vi "target_b2g2.vi"   [LabVIEW 2011]
uses:
  Output - Cluster b2g1.ctl
  Output - Cluster b2g2.ctl
  Input - Cluster b2g2.ctl
  <vilib>/Platform/TimedLoop/XDataNode/timing_clust.ctl
  <vilib>/Platform/TimedLoop/XDataNode/nitl_modes.ctl
  <vilib>/Platform/TimedLoop/XDataNode/wakeup.ctl
  <vilib>/Utility/error.llb/DialogType.ctl
  <vilib>/Platform/TimedLoop/XDataNode/XDataNode.xnode
  <vilib>/Platform/TimedLoop/XDataNode/XDNodeRunTimeDep.lvlib
panel:
  # "The Network Variable Engine and Variable Client Support must be installed on the RT target\nfor this application to function properly. If the Network Variable Engine is not supported on\nthe target (e.g.  FP-2000 with <32MB of RAM), open the project and move the variable library\nto My Computer in the project. Doing this will deploy the variables to localhost but\nwill still require that Variable Client Support be installed on the RT target."
types:
  T1 = typedef "XDNodeRunTimeDep.lvlib/timing_clust.ctl" = cluster{"Expected End [f-1]":u64, "Actual End [f-1]":u64, "Finished Late? [f-1]":bool, "Expected End [i-1]":u64, "Actual End [i-1]":u64, "Finished Late? [i-1]":bool, "Expected Start [i]":u64, "Actual Start [i]":u64, "Expected Start [f]":u64, "Actual Start [f]":u64, "Source Name":string, "Structure Name":string, "Period":i64, "Deadline":i64, "Offset":i64, "Start":i64, "Priority":i32, "Timeout":i32, "Mode":T2, "Wakeup Reason":T3, "Error":errorcluster, "Source Type":string, "Secondary Source Type":string, "Global End Time":u64, "Global Start Time":u64, "Frame Duration":u64, "Iteration Duration":u64, "Assigned CPU":i32, "I/O Scan Engine Mode":u32}
  T2 = typedef "XDNodeRunTimeDep.lvlib/nitl_modes.ctl" = enum32{"No Change", "Process missed periods, maintain original phase", "Discard missed periods, maintain original phase", "Process missed periods, ignore original phase", "Discard missed periods, ignore original phase"}
  T3 = typedef "XDNodeRunTimeDep.lvlib/wakeup.ctl" = enum32{"Normal", "Aborted", "Asynchronous wakeup", "Timing source error", "Timed loop error", "Timeout"}
  T4 = typedef "Output - Cluster b2g1.ctl" = cluster{"DFS-1 [dl]":u64, "FS-3 [l]":dbl, "DFS-1 [l/min]":dbl, "DS-1 [bar]":dbl, "V-10 ZU":bool, "V-14 ZU":bool, "FS-1 [l]":dbl, "FS-2 [l]":dbl, "TS-4 [°C]":dbl, "HS-1":bool, "V-13 [%]":u8, "V-15 [%]":u8, "P-4 [%]":u8, "P-5 [%]":u8, "Dosierung":bool, "MR Max Füllstand":bool, "MR Min Füllstand":bool, "Dosiermenge [l]":sgl, "V-14 AUF":bool, "V-10 AUF":bool, "T-1 Max Füllstand":bool, "T-1 Min Füllstand":bool, "T-2 Max Füllstand":bool, "T-2 Min Füllstand":bool, "pHS-1 [pH]":dbl, "P-4 RUN":bool, "P-5 RUN ":bool, "V-33 AUF":bool, "V-33 ZU":bool, "V-34 AUF":bool, "V-34 ZU":bool, "P-4 ERR":bool, "P-5 ERR":bool, "TS-5 [°C]":dbl, "TS-6 [°C]":dbl, "P-9 RUN":bool}
  T5 = cluster{"clusterb2g1":bool, "STOP":bool, "data - network -  b2g1":refnum<k21>, "shared variable refnum out":refnum<k21>}
  T6 = typedef "Output - Cluster b2g2.ctl" = cluster{"DFS-1 [dl]":u64, "FS-3 [l]":dbl, "DFS-1 [l/min]":dbl, "DS-1 [bar]":dbl, "V-10 ZU":bool, "V-14 ZU":bool, "FS-1 [l]":dbl, "FS-2 [l]":dbl, "TS-4 [°C]":dbl, "HS-1":bool, "V-13 [%]":u8, "V-15 [%]":u8, "P-4 [%]":u8, "Dosierung":bool, "MR Max Füllstand":bool, "MR Min Füllstand":bool, "Dosiermenge [l]":sgl, "V-14 AUF":bool, "V-10 AUF":bool, "T-1 Max Füllstand":bool, "T-1 Min Füllstand":bool, "T-2 Max Füllstand":bool, "T-2 Min Füllstand":bool, "pHS-1 [pH]":dbl, "P-4 RUN":bool, "V-33 AUF":bool, "V-33 ZU":bool, "V-34 AUF":bool, "V-34 ZU":bool, "P-4 ERR":bool, "TS-5 [°C]":dbl, "V-35 AUF":bool, "V-35 ZU":bool, "P-9 RUN":bool}
  T7 = cluster{"Durchflussregelung":dbl, "Temperaturregelung":bool, "STOP":bool, "Zirkulation":u64, "Dosierung Zeit":u64}
  T8 = typedef "Input - Cluster b2g2.ctl" = cluster{"V-13 [%]":u8, "V-15 [%]":u8, "Log-Target":bool, "P-4":bool, "P-4 Drehzahl [%]":u8, "Temperaturregelung":bool, "Überdruckregelung":bool, "Füllstandsregulierung":bool, "V-10":bool, "Log-Host":bool, "V-14":bool, "HS-1":bool, "Füllstand  P":sgl, "Füllstand I":sgl, "Füllstand D":sgl, "Füllstand Soll [l]":sgl, "Druck  P":sgl, "Druck I":sgl, "Druck D":sgl, "Druck Soll [bar]":sgl, "Temp Soll [°C]":sgl, "Dosierung":bool, "Dosiermenge [l]":sgl, "Dosiergeschw. [l/min]":sgl, "Tank":bool, "Hysterese [°C]":sgl, "MR Füllstandsüberwachung":bool, "Tank Füllstandsüberwachung":bool, "Log Target [ms]":u32, "Log Host [s]":u32, "Zirkulation EIN [min]":u8, "Zirkulation AUS [min]":u8, "Zirkulation":bool, "V-33":bool, "V-34":bool, "V-35":bool, "T1 Max Füllstand":bool, "T1 Min Füllstand":bool, "FS-1 [l]":sgl, "P-9":bool}
  T9 = typedef "DialogType.ctl" = u16
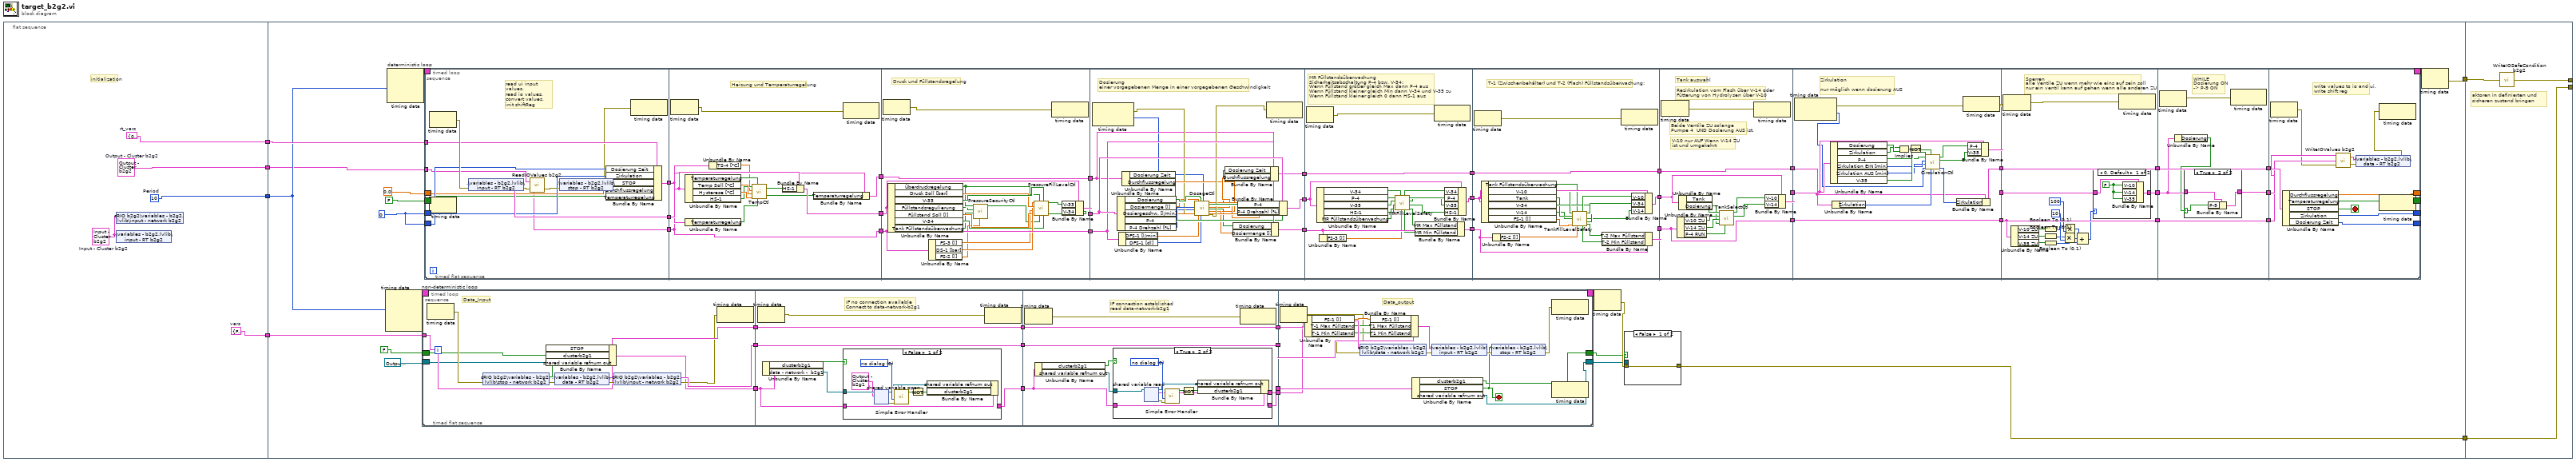
[diagram p0: block diagram]
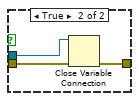
[diagram p2: hidden frame]
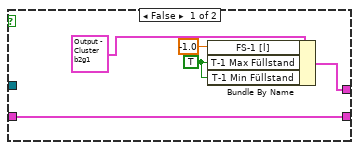
[diagram p4: hidden frame]
diagram:
  n1 = flat-sequence {
    tunnel: [w10] -> w6
    tunnel: [w9] -> w5
    tunnel: [w8] -> w4
    tunnel: [w7] -> w1
    tunnel: w6 -> [w23]
    tunnel: w5 -> [w22]
    tunnel: w4 -> [w21]
    tunnel: [w17] -> w3
    tunnel: [w20] -> w2
    tunnel: w1 -> [w16]
    tunnel: w3 -> [w441]
    tunnel: w2 -> [w440]
    tunnel: [w439] -> _
    tunnel: [w441] -> _
    frame #0 {
      w7 = T5 {"clusterb2g1"=FALSE, "STOP"=FALSE, "data - network -  b2g1"="ni.var.psp://10.27.40.24/variables - b2g1/data - network - b2g1", "shared variable refnum out"=""}  # vars
      w8 = T6 {"DFS-1 [dl]"=0, "FS-3 [l]"=0.0, "DFS-1 [l/min]"=0.0, "DS-1 [bar]"=0.0, "V-10 ZU"=FALSE, "V-14 ZU"=FALSE, "FS-1 [l]"=0.0, "FS-2 [l]"=0.0, "TS-4 [°C]"=0.0, "HS-1"=FALSE, "V-13 [%]"=0, "V-15 [%]"=0, "P-4 [%]"=0, "Dosierung"=FALSE, "MR Max Füllstand"=FALSE, "MR Min Füllstand"=FALSE, "Dosiermenge [l]"=0.0, "V-14 AUF"=FALSE, "V-10 AUF"=FALSE, "T-1 Max Füllstand"=FALSE, "T-1 Min Füllstand"=FALSE, "T-2 Max Füllstand"=FALSE, "T-2 Min Füllstand"=FALSE, "pHS-1 [pH]"=0.0, "P-4 RUN"=FALSE, "V-33 AUF"=FALSE, "V-33 ZU"=FALSE, "V-34 AUF"=FALSE, "V-34 ZU"=FALSE, "P-4 ERR"=FALSE, "TS-5 [°C]"=0.0, "V-35 AUF"=FALSE, "V-35 ZU"=FALSE, "P-9 RUN"=FALSE}  # Output - Cluster b2g2
      w10 = T7 {"Durchflussregelung"=0.0, "Temperaturregelung"=FALSE, "STOP"=FALSE, "Zirkulation"=0, "Dosierung Zeit"=0}  # rt_vars
      w9 = i64 10  # Period
      w11 = T8 {"V-13 [%]"=0, "V-15 [%]"=0, "Log-Target"=FALSE, "P-4"=FALSE, "P-4 Drehzahl [%]"=0, "Temperaturregelung"=FALSE, "Überdruckregelung"=FALSE, "Füllstandsregulierung"=FALSE, "V-10"=FALSE, "Log-Host"=FALSE, "V-14"=FALSE, "HS-1"=FALSE, "Füllstand  P"=0.0, "Füllstand I"=0.0, "Füllstand D"=0.0, "Füllstand Soll [l]"=0.0, "Druck  P"=0.0, "Druck I"=0.0, "Druck D"=0.0, "Druck Soll [bar]"=0.0, "Temp Soll [°C]"=0.0, "Dosierung"=FALSE, "Dosiermenge [l]"=0.0, "Dosiergeschw. [l/min]"=0.0, "Tank"=FALSE, "Hysterese [°C]"=0.0, "MR Füllstandsüberwachung"=FALSE, "Tank Füllstandsüberwachung"=FALSE, "Log Target [ms]"=0, "Log Host [s]"=0, "Zirkulation EIN [min]"=0, "Zirkulation AUS [min]"=0, "Zirkulation"=FALSE, "V-33"=FALSE, "V-34"=FALSE, "V-35"=FALSE, "T1 Max Füllstand"=FALSE, "T1 Min Füllstand"=FALSE, "FS-1 [l]"=0.0, "P-9"=FALSE}  # Input - Cluster b2g2
      # "initialization"
      n2 = shared-variable "cRIO b2g2\\variables - b2g2.lvlib\\input - network b2g2"(w11) -> ()  [unwired: 1 in, 1 out]
      n3 = shared-variable ".\\variables - b2g2.lvlib\\input - RT b2g2"(w11) -> ()  [unwired: 1 in, 1 out]
    }
    frame #1 {
      w19 = u64 0
      n4 = node-c288 ("Input Node")(w22) -> (w27:T1)  [unwired: 3 in]
      n5 = node-c288 ("Input Node")(w22) -> (w29:T1)  [unwired: 2 in]
      n6 = timed-loop "non-deterministic loop" {
        timing: w27 -> [_]
        timing-out: [_] -> w26
        tunnel: w16 -> [w38]
        shift-right: [w37] -> w12
        shift-left: FALSE ("stop - network b2g2") -> [w36]
        shift-right: [w35] -> w13
        shift-left: refnum<k21> refnum ("shared variable refnum out") -> [w34]
        stop <- w123 stop-if-true
        n7 = timed-sequence {
          timing: _ -> [_]
          timing-out: _ -> [_]
          tunnel: w38 -> [w50]
          tunnel: [w49] -> w37
          tunnel: w36 -> [w48]
          tunnel: [w40] -> w35
          tunnel: w34 -> [w39]
          n8 = timed-flat-sequence {
            tunnel: [w63] -> w52
            tunnel: [w62] -> w53
            tunnel: [w57] -> w51
            tunnel: w50 -> [w58]
            tunnel: w48 -> [w55]
            tunnel: w39 -> [w54]
            tunnel: w53 -> [w76]
            tunnel: [w76] -> w47
            tunnel: w52 -> [w75]
            tunnel: [w75] -> w45
            tunnel: w51 -> [w72]
            tunnel: [w71] -> w43
            tunnel: w47 -> [w99]
            tunnel: [w99] -> w46
            tunnel: w45 -> [w98]
            tunnel: [w98] -> w44
            tunnel: w43 -> [w96]
            tunnel: [w95] -> w42
            tunnel: [w93] -> w41
            tunnel: w46 -> [w129]
            tunnel: w44 -> [w130]
            tunnel: w42 -> [w124]
            tunnel: [w122] -> w49
            tunnel: w41 -> [w121]
            tunnel: [w119] -> w40
            frame #0 {
              # "Data_Input"
              n9 = node-c288() -> (w61:errorcluster)  [unwired: 1 in]
              n10 = shared-variable "cRIO b2g2\\variables - b2g2.lvlib\\stop - network b2g2"(error in=w61) -> (w56:bool, error out=w60:errorcluster)
              n11 = Bundle By Name(cluster=w58, "STOP"=w56, "clusterb2g1"=w55, "shared variable refnum out"=w54) -> (w57:T5)
              n12 = shared-variable ".\\variables - b2g2.lvlib\\data - RT b2g2"(error in=w60) -> (w63:T6, error out=w64:errorcluster)
              n13 = shared-variable "cRIO b2g2\\variables - b2g2.lvlib\\input - network b2g2"(error in=w64) -> (w62:T8, error out=w59:errorcluster)
              n14 = node-c288(w59) -> ()  [unwired: 1 out]
            }
            frame #1 {
              # "IF no connection available\nConnect to data-network-b2g1"
              n15 = node-c288() -> (w70:errorcluster)  [unwired: 1 in]
              n16 = Unbundle By Name(w72) -> ("clusterb2g1"=w73:bool, "data - network -  b2g1"=w74:refnum<k21>)
              n17 = case shown="False" w73 {
                tunnel: w74 -> [w85 _]
                tunnel: [w79 w86] -> w71
                tunnel: w72 -> [w80 w86]
                frame False {
                  w83 = T9 0 items=["no dialog", "OK message", "continue or stop message", "OK message + warnings", "continue/stop + warnings"] ("type of dialog (OK msg:1)")
                  n18 = shared-variable-open(w85, T4 {"DFS-1 [dl]"=0, "FS-3 [l]"=0.0, "DFS-1 [l/min]"=0.0, "DS-1 [bar]"=0.0, "V-10 ZU"=FALSE, "V-14 ZU"=FALSE, "FS-1 [l]"=0.0, "FS-2 [l]"=0.0, "TS-4 [°C]"=0.0, "HS-1"=FALSE, "V-13 [%]"=0, "V-15 [%]"=0, "P-4 [%]"=0, "P-5 [%]"=0, "Dosierung"=FALSE, "MR Max Füllstand"=FALSE, "MR Min Füllstand"=FALSE, "Dosiermenge [l]"=0.0, "V-14 AUF"=FALSE, "V-10 AUF"=FALSE, "T-1 Max Füllstand"=FALSE, "T-1 Min Füllstand"=FALSE, "T-2 Max Füllstand"=FALSE, "T-2 Min Füllstand"=FALSE, "pHS-1 [pH]"=0.0, "P-4 RUN"=FALSE, "P-5 RUN "=FALSE, "V-33 AUF"=FALSE, "V-33 ZU"=FALSE, "V-34 AUF"=FALSE, "V-34 ZU"=FALSE, "P-4 ERR"=FALSE, "P-5 ERR"=FALSE, "TS-5 [°C]"=0.0, "TS-6 [°C]"=0.0, "P-9 RUN"=FALSE} ("Output - Cluster b2g1")) -> (w77:refnum<k21>, w82:errorcluster)  [unwired: 2 in]
                  n19 = call <vilib>:"Simple Error Handler.vi"("type of dialog (OK msg:1)"=w83, "error in (no error)"=w82) -> ("error?"=w81:bool)  [unwired: 3 in, 4 out]
                  n20 = Not(x=w81) -> (.not. x?=w78:bool)
                  n21 = Bundle By Name(cluster=w80, "shared variable refnum out"=w77, "clusterb2g1"=w78) -> (w79:T5)
                }
                frame True {
                }
              }
              n22 = node-c288(w70) -> ()  [unwired: 1 out]
            }
            frame #2 {
              # "IF connection established\nread data-network-b2g1"
              n23 = node-c288() -> (w92:errorcluster)  [unwired: 1 in]
              n24 = Unbundle By Name(w96) -> ("clusterb2g1"=w97:bool, "shared variable refnum out"=w94:refnum<k21>)
              n25 = case shown="True" w97 {
                tunnel: w94 -> [_ w108]
                tunnel: [w104 w110] -> w95
                tunnel: w96 -> [w104 w111]
                tunnel: [w103 w105] -> w93
                frame False {
                  w101 = TRUE ("T-1 Max Füllstand")
                  n26 = Bundle By Name(cluster=T4 {"DFS-1 [dl]"=0, "FS-3 [l]"=0.0, "DFS-1 [l/min]"=0.0, "DS-1 [bar]"=0.0, "V-10 ZU"=FALSE, "V-14 ZU"=FALSE, "FS-1 [l]"=0.0, "FS-2 [l]"=0.0, "TS-4 [°C]"=0.0, "HS-1"=FALSE, "V-13 [%]"=0, "V-15 [%]"=0, "P-4 [%]"=0, "P-5 [%]"=0, "Dosierung"=FALSE, "MR Max Füllstand"=FALSE, "MR Min Füllstand"=FALSE, "Dosiermenge [l]"=0.0, "V-14 AUF"=FALSE, "V-10 AUF"=FALSE, "T-1 Max Füllstand"=FALSE, "T-1 Min Füllstand"=FALSE, "T-2 Max Füllstand"=FALSE, "T-2 Min Füllstand"=FALSE, "pHS-1 [pH]"=0.0, "P-4 RUN"=FALSE, "P-5 RUN "=FALSE, "V-33 AUF"=FALSE, "V-33 ZU"=FALSE, "V-34 AUF"=FALSE, "V-34 ZU"=FALSE, "P-4 ERR"=FALSE, "P-5 ERR"=FALSE, "TS-5 [°C]"=0.0, "TS-6 [°C]"=0.0, "P-9 RUN"=FALSE} ("Output - Cluster b2g1"), "FS-1 [l]"=-1.0, "T-1 Max Füllstand"=w101, "T-1 Min Füllstand"=w101) -> (w103:T4)
                }
                frame True {
                  w113 = T9 0 items=["no dialog", "OK message", "continue or stop message", "OK message + warnings", "continue/stop + warnings"] ("type of dialog (OK msg:1)")
                  n27 = shared-variable-read(w108) -> (w106:refnum<k21>, w107:errorcluster, w105:T4)  [unwired: 1 in, 1 out]
                  n28 = call <vilib>:"Simple Error Handler.vi"("type of dialog (OK msg:1)"=w113, "error in (no error)"=w107) -> ("error?"=w112:bool)  [unwired: 3 in, 4 out]
                  n29 = Not(x=w112) -> (.not. x?=w109:bool)
                  n30 = Bundle By Name(cluster=w111, "shared variable refnum out"=w106, "clusterb2g1"=w109) -> (w110:T5)
                }
              }
              n31 = node-c288(w92) -> ()  [unwired: 1 out]
            }
            frame #3 {
              # "Data_output"
              n32 = node-c288() -> (w120:errorcluster)  [unwired: 1 in]
              n33 = Unbundle By Name(w121) -> ("FS-1 [l]"=w125:dbl, "T-1 Max Füllstand"=w127:bool, "T-1 Min Füllstand"=w126:bool)
              n34 = shared-variable "cRIO b2g2\\variables - b2g2.lvlib\\data - network b2g2"(w130, error in=w120) -> (error out=w133:errorcluster)
              n35 = Bundle By Name(cluster=w129, "FS-1 [l]"=w125, "T1 Max Füllstand"=w127, "T1 Min Füllstand"=w126) -> (w128:T8)
              n36 = Unbundle By Name(w124) -> ("clusterb2g1"=w122:bool, "STOP"=w123:bool, "shared variable refnum out"=w119:refnum<k21>)
              n37 = shared-variable ".\\variables - b2g2.lvlib\\input - RT b2g2"(w128, error in=w133) -> (error out=w132:errorcluster)
              n38 = shared-variable ".\\variables - b2g2.lvlib\\stop - RT b2g2"(w123, error in=w132) -> (error out=w131:errorcluster)
              n39 = node-c288(w131) -> ()  [unwired: 1 out]
            }
          }
        }
        n40 = node-c288() -> ()  [unwired: 1 in, 1 out]
        n41 = node-c288() -> ()  [unwired: 1 in, 1 out]
      }
      n42 = timed-loop "deterministic loop" {
        timing: w29 -> [_]
        timing-out: [_] -> w28
        shift-right: [w155] -> _
        shift-left: 0.0 -> [w154]
        shift-right: [w153] -> _
        shift-left: FALSE ("Temperaturregelung") -> [w151]
        tunnel: w23 -> [w152]
        tunnel: w21 -> [w150]
        shift-right: [w149] -> _
        shift-left: w19 -> [w148]
        shift-right: [w147] -> _
        shift-left: w19 -> [w146]
        stop <- w422 stop-if-true
        n43 = timed-sequence {
          timing: _ -> [_]
          timing-out: _ -> [_]
          tunnel: [w193] -> w155
          tunnel: w154 -> [w192]
          tunnel: [w189] -> w153
          tunnel: w152 -> [w188]
          tunnel: w151 -> [w186]
          tunnel: w150 -> [w181]
          tunnel: [w174] -> w149
          tunnel: w148 -> [w173]
          tunnel: [w172] -> w147
          tunnel: w146 -> [w171]
          n44 = timed-flat-sequence {
            tunnel: [w209] -> w191
            tunnel: [w199] -> w190
            tunnel: w192 -> [w202]
            tunnel: w188 -> [w207]
            tunnel: [w206] -> w187
            tunnel: w186 -> [w201]
            tunnel: w181 -> [w200]
            tunnel: w173 -> [w205]
            tunnel: w171 -> [w204]
            tunnel: w191 -> [w224]
            tunnel: w190 -> [w216]
            tunnel: [w216] -> w167
            tunnel: w187 -> [w220]
            tunnel: [w221] -> w166
            tunnel: [w223] -> w165
            tunnel: [w249] -> w195
            tunnel: w167 -> [w247]
            tunnel: [w247] -> w194
            tunnel: w166 -> [w251]
            tunnel: [w251] -> w185
            tunnel: w165 -> [w248]
            tunnel: w195 -> [w280]
            tunnel: [w278] -> w180
            tunnel: w194 -> [w279]
            tunnel: [w273] -> w179
            tunnel: w185 -> [w265]
            tunnel: [w269] -> w178
            tunnel: w180 -> [w293]
            tunnel: [w292] -> w184
            tunnel: w179 -> [w302]
            tunnel: [w301] -> w183
            tunnel: w178 -> [w304]
            tunnel: [w304] -> w182
            tunnel: w184 -> [w317]
            tunnel: [w318] -> w177
            tunnel: w183 -> [w325]
            tunnel: [w324] -> w176
            tunnel: w182 -> [w327]
            tunnel: [w327] -> w175
            tunnel: w177 -> [w336]
            tunnel: [w337] -> w164
            tunnel: w176 -> [w341]
            tunnel: [w341] -> w163
            tunnel: w175 -> [w344]
            tunnel: [w344] -> w162
            tunnel: [w357] -> w170
            tunnel: [w368] -> w169
            tunnel: [w358] -> w168
            tunnel: w164 -> [w356]
            tunnel: w163 -> [w368]
            tunnel: w162 -> [w359]
            tunnel: w170 -> [w376]
            tunnel: [w375] -> w161
            tunnel: w169 -> [w388]
            tunnel: [w388] -> w159
            tunnel: w168 -> [w390]
            tunnel: [w390] -> w157
            tunnel: w161 -> [w401]
            tunnel: [w403] -> w160
            tunnel: w159 -> [w402]
            tunnel: [w402] -> w158
            tunnel: w157 -> [w405]
            tunnel: [w405] -> w156
            tunnel: w160 -> [w419]
            tunnel: w158 -> [w418]
            tunnel: [w423] -> w193
            tunnel: [w424] -> w189
            tunnel: w156 -> [w425]
            tunnel: [w421] -> w174
            tunnel: [w420] -> w172
            frame #0 {
              # "read ui input values,\nread io values,\nconvert values,\ninit shiftReg"
              n45 = node-c288 ("Output Node")() -> (w208:errorcluster)  [unwired: 1 in]
              n46 = shared-variable ".\\variables - b2g2.lvlib\\input - RT b2g2"(error in=w208) -> (w209:T8, error out=w198:errorcluster)
              n47 = call "ReadIOValues b2g2.vi"("error in"=w198, "Output - Cluster b2g2 2"=w200) -> ("error out"=w197:errorcluster, "Output - Cluster b2g2"=w199:T6)
              n48 = shared-variable ".\\variables - b2g2.lvlib\\stop - RT b2g2"(error in=w197) -> (w203:bool, error out=w196:errorcluster)
              n49 = Bundle By Name(cluster=w207, "Dosierung Zeit"=w204, "Zirkulation"=w205, "STOP"=w203, "Durchflussregelung"=w202, "Temperaturregelung"=w201) -> (w206:T7)
              n50 = node-c288 ("Input Node")(w196) -> ()  [unwired: 1 out]
            }
            frame #1 {
              # "Heizung und Temperaturregelung"
              n51 = node-c288() -> (w228:errorcluster)  [unwired: 1 in]
              n52 = Unbundle By Name(w224) -> ("Temperaturregelung"=w227:bool, "Temp Soll [°C]"=w226:sgl, "Hysterese [°C]"=w225:sgl, "HS-1"=w217:bool)
              n53 = Unbundle By Name(w220) -> ("Temperaturregelung"=w219:bool)
              n54 = Unbundle By Name(w216) -> ("TS-4 [°C]"=w215:dbl)
              n55 = call "TempCtl.vi"("shiftReg"=w219, "enable"=w227, "Hysterese"=w225, "Soll"=w226, "IST"=w215, "heating"=w217) -> ("shiftReg"=w218:bool, "heating"=w222:bool)
              n56 = Bundle By Name(cluster=w224, "HS-1"=w222) -> (w223:T8)
              n57 = Bundle By Name(cluster=w220, "Temperaturregelung"=w218) -> (w221:T7)
              n58 = node-c288(w228) -> ()  [unwired: 1 out]
            }
            frame #2 {
              # "Druck und Füllstandsregelung"
              n59 = node-c288() -> (w250:errorcluster)  [unwired: 1 in]
              n60 = Unbundle By Name(w248) -> ("Überdruckregelung"=w237:bool, "Druck Soll [bar]"=w245:sgl, "V-33"=w246:bool, "Füllstandsregulierung"=w236:bool, "Füllstand Soll [l]"=w242:sgl, "V-34"=w243:bool, "Tank Füllstandsüberwachung"=w235:bool)
              n61 = Unbundle By Name(w247) -> ("FS-3 [l]"=w241:dbl, "DS-1 [bar]"=w244:dbl, "FS-2 [l]"=w238:dbl)
              n62 = call "PressureSecurityCtl.vi"("FS-2 [l]"=w238, "Tank Füllstandsüberwachung"=w235, "Füllstandsregulierung"=w236, "Überdruckregelung"=w237) -> ("Füllstandsregulierung"=w234:bool)  [unwired: 7 in]
              n63 = call "PressureFillLevelCtl.vi"("LiquidValve"=w243, "GasValve"=w246, "FillLevelCtl"=w234, "PressureCtl"=w237, "V_setpoint"=w242, "V_value"=w241, "P_setpoint"=w245, "P_value"=w244) -> ("LiquidValve"=w239:bool, "GasValve"=w240:bool)  [unwired: 2 in]
              n64 = node-c288(w250) -> ()  [unwired: 1 out]
              n65 = Bundle By Name(cluster=w248, "V-33"=w240, "V-34"=w239) -> (w249:T8)
            }
            frame #3 {
              # "Dosierung \neiner vorgegebenen Menge in einer vorgegebenen Geschwindigkeit"
              n66 = node-c288() -> (w266:errorcluster, w260:i64)  [unwired: 1 in]
              n67 = Unbundle By Name(w280) -> ("Dosierung"=w271:bool, "Dosiermenge [l]"=w257:sgl, "Dosiergeschw. [l/min]"=w274:sgl, "P-4"=w277:bool, "P-4 Drehzahl [%]"=w276:u8)
              n68 = Unbundle By Name(w279) -> ("DFS-1 [l/min]"=w262:dbl, "DFS-1 [dl]"=w263:u64)
              n69 = Unbundle By Name(w265) -> ("Dosierung Zeit"=w261:u64, "Durchflussregelung"=w267:dbl)
              n70 = call "DosageCtl.vi"("setpoint volume flow [l/min]"=w274, "pump"=w277, "value speed [%]"=w276, "shiftReg int"=w261, "shiftReg dbl"=w267, "error in (no error)"=w266, "setpoint volume [l]"=w257, "value volume flow [l/min]"=w262, "enable"=w271, "value volume [dl]"=w263, "Actual Start [f]"=w260) -> ("pump"=w264:bool, "speed [%]"=w272:dbl, "shiftReg int"=w259:u64, "shiftreg dbl"=w268:dbl, "enable"=w258:bool, "volume[l]"=w270:dbl, "error out"=w275:errorcluster)  [unwired: 2 in]
              n71 = Bundle By Name(cluster=w265, "Dosierung Zeit"=w259, "Durchflussregelung"=w268) -> (w269:T7)
              n72 = Bundle By Name(cluster=w279, "Dosierung"=w258, "Dosiermenge [l]"=w270) -> (w273:T6)
              n73 = Bundle By Name(cluster=w280, "P-4"=w264, "P-4 Drehzahl [%]"=w272) -> (w278:T8)
              n74 = node-c288(w275) -> ()  [unwired: 1 out]
            }
            frame #4 {
              # "MR Füllstandsüberwachung\nSicherheitsabschaltung P-4 bzw. V-34:\nWenn Füllstand größer gleich Max dann P-4 aus\nWenn Füllstand kleiner gleich Min dann V-34 und V-35 zu\nWenn Füllstand kleiner gleich 0 dann HS-1 aus"
              n75 = node-c288() -> (w303:errorcluster)  [unwired: 1 in]
              n76 = Unbundle By Name(w293) -> ("V-34"=w297:bool, "P-4"=w296:bool, "V-35"=w295:bool, "HS-1"=w294:bool, "MR Füllstandsüberwachung"=w288:bool)
              n77 = Unbundle By Name(w302) -> ("FS-3 [l]"=w298:dbl)
              n78 = call "MRFillLevelSafety.vi"("fill level [l]"=w298, "Valve"=w297, "enable"=w288, "Heating"=w294, "Circulation"=w295, "Pump"=w296) -> ("max level"=w300:bool, "Heating"=w289:bool, "Circulation"=w287:bool, "Pump"=w290:bool, "min level"=w299:bool, "Valve"=w291:bool)
              n79 = Bundle By Name(cluster=w302, "MR Max Füllstand"=w300, "MR Min Füllstand"=w299) -> (w301:T6)
              n80 = node-c288(w303) -> ()  [unwired: 1 out]
              n81 = Bundle By Name(cluster=w293, "V-34"=w291, "P-4"=w290, "V-35"=w287, "HS-1"=w289) -> (w292:T8)
            }
            frame #5 {
              # "T-1 (Zwischenbehälter) und T-2 (Flash) Füllstandsüberwachung:"
              n82 = node-c288() -> (w326:errorcluster)  [unwired: 1 in]
              n83 = Unbundle By Name(w317) -> ("Tank Füllstandsüberwachung"=w313:bool, "V-10"=w316:bool, "Tank"=w314:bool, "V-34"=w315:bool, "V-14"=w312:bool, "FS-1 [l]"=w310:sgl)
              n84 = Unbundle By Name(w325) -> ("FS-2 [l]"=w322:dbl)
              n85 = call "TankFillLevelSafety.vi"("pump"=w316, "enable"=w313, "tank"=w314, "intlet valve"=w312, "outlet valve"=w315, "fill level t-1"=w310, "fill level t-2"=w322) -> ("pump"=w320:bool, "outlet valve"=w319:bool, "inlet valve"=w311:bool, "min level t-2"=w323:bool, "max level t-2"=w321:bool)  [unwired: 2 in, 2 out]
              n86 = Bundle By Name(cluster=w325, "T-2 Max Füllstand"=w321, "T-2 Min Füllstand"=w323) -> (w324:T6)
              n87 = node-c288(w326) -> ()  [unwired: 1 out]
              n88 = Bundle By Name(cluster=w317, "V-10"=w320, "V-34"=w319, "V-14"=w311) -> (w318:T8)
            }
            frame #6 {
              # "V-10 nur AUF Wenn V-14 ZU\nist und umgekehrt"
              # "Beide Ventile ZU solange \nPumpe 4  UND Dosierung AUS ist."
              # "Rezirkulation vom Flash über V-14 oder \nFütterung von Hydrolysen über V-10"
              # "Tank auswahl"
              n89 = node-c288() -> (w342:errorcluster)  [unwired: 1 in]
              n90 = Unbundle By Name(w341) -> ("V-10 ZU"=w339:bool, "V-14 ZU"=w340:bool, "P-4 RUN"=w338:bool)
              n91 = Unbundle By Name(w336) -> ("Tank"=w343:bool, "Dosierung"=w333:bool)
              n92 = call "TankSelectCtl.vi"("pump"=w338, "enable"=w333, "valve t-2 close"=w340, "valve t-1 close"=w339, "Tank"=w343) -> ("valve t-2"=w334:bool, "valve t-1"=w335:bool)  [unwired: 5 in]
              n93 = node-c288(w342) -> ()  [unwired: 1 out]
              n94 = Bundle By Name(cluster=w336, "V-10"=w335, "V-14"=w334) -> (w337:T8)
            }
            frame #7 {
              # "Zirkulation\n\nnur möglich wenn dosierung AUS"
              n95 = node-c288() -> (w350:errorcluster, w351:i64)  [unwired: 1 in]
              n96 = Unbundle By Name(w356) -> ("Dosierung"=w354:bool, "Zirkulation"=w353:bool, "P-4"=w362:bool, "Zirkulation EIN [min]"=w361:u8, "Zirkulation AUS [min]"=w360:u8, "V-35"=w363:bool)
              n97 = Unbundle By Name(w359) -> ("Zirkulation"=w364:u64)
              n98 = Implies(1:w354, 2:w353) -> (0:w355:bool)
              n99 = Not(x=w355) -> (.not. x?=w352:bool)
              n100 = call "CirculationCtl.vi"("Valve"=w363, "shiftReg[ms]"=w364, "enable"=w352, "Actual Start [ms]"=w351, "OffTime [min]"=w360, "OnTime [min]"=w361, "Pump"=w362) -> ("shiftReg[ms]"=w365:u64, "Valve"=w366:bool, "Pump"=w367:bool)  [unwired: 2 in]
              n101 = Bundle By Name(cluster=w359, "Zirkulation"=w365) -> (w358:T7)
              n102 = node-c288(w350) -> ()  [unwired: 1 out]
              n103 = Bundle By Name(cluster=w356, "P-4"=w367, "V-35"=w366) -> (w357:T8)
            }
            frame #8 {
              # "Sperren\nalle Ventile ZU wenn mehr wie eins auf sein soll\nnur ein ventil kann auf gehen wenn alle anderen ZU"
              n104 = node-c288() -> (w389:errorcluster)  [unwired: 1 in]
              n105 = Unbundle By Name(w388) -> ("V-10 ZU"=w387:bool, "V-14 ZU"=w386:bool, "V-35 ZU"=w385:bool)
              n106 = Boolean To (0,1)(Boolean=w387) -> (0, 1=w377:i16)
              n107 = Boolean To (0,1)(Boolean=w386) -> (0, 1=w381:i16)
              n108 = Boolean To (0,1)(Boolean=w385) -> (0, 1=w383:i16)
              n109 = Multiply(x=w381, y=i16 10) -> (x*y=w380:i16)
              n110 = Multiply(x=w377, y=i16 100) -> (x*y=w379:i16)
              n111 = Compound Arithmetic op=ADD(w379, w380, w383) -> (w384:i16)
              n112 = case shown="0, Default" w384 {
                tunnel: w376 -> [w393 w394]
                tunnel: [w392 w394] -> w375
                frame 0, Default {
                  w391 = FALSE ("V-10")
                  n113 = Bundle By Name(cluster=w393, "V-10"=w391, "V-14"=w391, "V-35"=w391) -> (w392:T8)
                }
                frame 11, 101, 110, 111 {
                }
              }
              n114 = node-c288(w389) -> ()  [unwired: 1 out]
            }
            frame #9 {
              # "WHILE\nDosierung ON\n-> P-9 ON"
              n115 = node-c288() -> (w404:errorcluster)  [unwired: 1 in]
              n116 = Unbundle By Name(w401) -> ("Dosierung"=w400:bool)
              n117 = case shown="True" w400 {
                selector: w400 -> [_ w407]
                tunnel: w401 -> [w406 w409]
                tunnel: [w406 w408] -> w403
                frame False {
                }
                frame True {
                  n118 = Bundle By Name(cluster=w409, "P-9"=w407) -> (w408:T8)
                }
              }
              n119 = node-c288(w404) -> ()  [unwired: 1 out]
            }
            frame #10 {
              # "write values to io and ui,\nwrite shift reg"
              n120 = node-c288() -> (w416:errorcluster)  [unwired: 1 in]
              n121 = Unbundle By Name(w425) -> ("Durchflussregelung"=w423:dbl, "Temperaturregelung"=w424:bool, "STOP"=w422:bool, "Zirkulation"=w421:u64, "Dosierung Zeit"=w420:u64)
              n122 = call "WriteIOValues b2g2.vi"("error in"=w416, "Output - Cluster b2g2"=w418, "input cluster"=w419) -> ("error out"=w415:errorcluster, "output cluster"=w417:T6)
              n123 = shared-variable ".\\variables - b2g2.lvlib\\data - RT b2g2"(w417, error in=w415) -> (error out=w426:errorcluster)
              n124 = node-c288(w426) -> ()  [unwired: 1 out]
            }
          }
        }
        n125 = node-c288() -> ()  [unwired: 1 in, 1 out]
        n126 = node-c288() -> ()  [unwired: 1 in, 1 out]
      }
      n127 = node-c288 ("Output Node")(w26) -> (w18:errorcluster)
      n128 = case shown="False" w12 {
        tunnel: w18 -> [w30 w33]
        tunnel: [w30 w32] -> w17
        tunnel: w13 -> [_ w31]
        frame False {
        }
        frame True {
          n129 = Close Variable Connection(8:w33, 11:w31) -> (0:w32:errorcluster)
        }
      }
      n130 = node-c288 ("Output Node")(w28) -> (w20:errorcluster)
    }
    frame #2 {
      # "aktoren in definierten und sicheren zustand bringen"
      n131 = call "WriteIOSafeCondition b2g2.vi"("error in"=w440) -> ("error out"=w439:errorcluster)
    }
  }
